vi "Configure Math Function (FFT Characteristics).vi"(4 "Math Function Index (1: Math Function 1)":i32(ring)=1 items=["Math Function 1"=1, "Math Function 2"=2, "Math Function 3"=3, "Math Function 4"=4], 7 "Gate (0: None)":i32(ring) items=["None", "Zoom"], 8 "error in (no error)":errorcluster, 9 "Readout Type (0: Sample Rate)":i32(ring) items=["Sample Rate", "Bin Size", "Resolution Bandwidth"], 10 "Readout Index (1: Readout 1)":i32(ring)=1 items=["Readout 1"=1, "Readout 2"=2], 11 "VISA resource name":refnum<visa-resource-name>) -> (0 "error out":errorcluster, 3 "VISA resource name out":refnum<visa-resource-name>)   [LabVIEW 2015, in "Agilent 2000 3000 X-Series.lvlib"]
doc: "Configures the math function FFT characteristics.\n\n<b>Note:</b>\n - This VI is applicable for 3000T, 4000, 6000 Series."
uses:
  Agilent 2000 3000 X-Series.lvlib
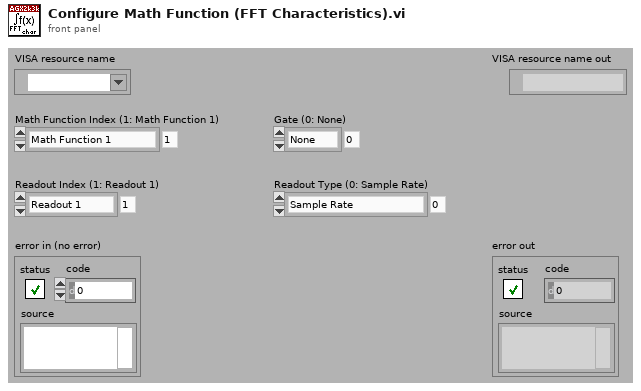
[diagram p1: front panel]
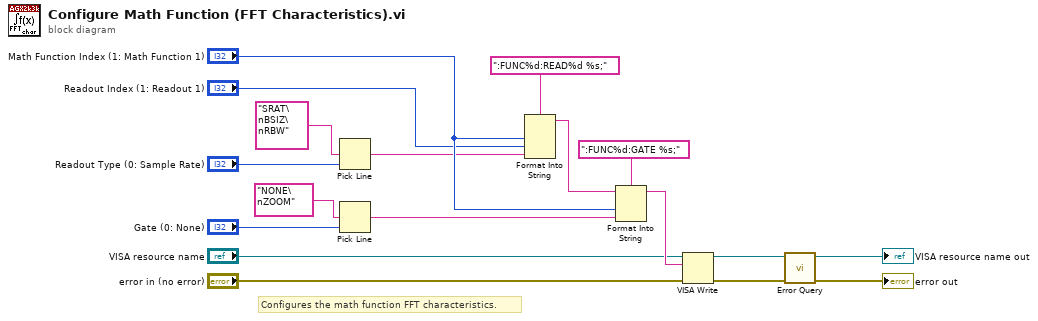
[diagram p0: block diagram]
diagram:
  # "Configures the math function FFT characteristics."
  n1 = Pick Line(multi-line string="SRAT\nBSIZ\nRBW", line index="Readout Type (0: Sample Rate)") -> (output string=w13:string)  [unwired: 1 in]
  n2 = Pick Line(multi-line string="NONE\nZOOM", line index="Gate (0: None)") -> (output string=w8:string)  [unwired: 1 in]
  n3 = Format Into String(format string=":FUNC%d:READ%d %s;", "Math Function Index (1: Math Function 1)", "Readout Index (1: Readout 1)", w13) -> (resulting string=w10:string)  [unwired: 2 in, 1 out]
  n4 = Format Into String(format string=":FUNC%d:GATE %s;", initial string=w10, "Math Function Index (1: Math Function 1)", w8) -> (resulting string=w7:string)  [unwired: 1 in, 1 out]
  n5 = VISA Write(VISA resource name="VISA resource name", write buffer=w7, error in (no error)="error in (no error)") -> (VISA resource name out=w4:refnum<visa-resource-name>, error out=w3:errorcluster)  [unwired: 1 out]
  n6 = call "Error Query.vi"("error in (no error)"=w3, "VISA resource name"=w4) -> ("error out"=→"error out":errorcluster, "VISA resource name out"=→"VISA resource name out":refnum<visa-resource-name>)  [unwired: 6 in, 2 out]
